vi "armctrl-arm-ctrl-exec.vi"(9 "Process Variable\nRadians":dbl, 10 "Setpoint Radians":dbl, 11 "in Linear System Loop":T1) -> (0 "Error":bool, 1 "Filtered Process\nVariable Radians":dbl, 2 "Motor Dmd":dbl, 3 "out Linear System Loop":T1)   [LabVIEW 2019]
uses:
  <vilib>/Rock Robotics/WPI/ThirdParty/JAS_Junk/TrajLib/TypeDef/LINEAR_SYSTEM_LOOP.ctl
  <vilib>/Rock Robotics/WPI/ThirdParty/JAS_Junk/TrajLib/TypeDef/LINEAR_QUADRATIC_REGULATOR.ctl
  <vilib>/Analysis/Matrix/Datatypes/RealMatrix.ctl
  <vilib>/Rock Robotics/WPI/ThirdParty/JAS_Junk/TrajLib/TypeDef/LINEAR_PLANT_INV_FF.ctl
  <vilib>/Rock Robotics/WPI/ThirdParty/JAS_Junk/TrajLib/TypeDef/KALMAN_FILTER.ctl
  <vilib>/Rock Robotics/WPI/ThirdParty/JAS_Junk/TrajLib/TypeDef/LINEAR_SYSTEM.ctl
  <vilib>/Rock Robotics/WPI/ThirdParty/JAS_Junk/TrajLib/MatBuilder_Create.vi
  <vilib>/Rock Robotics/WPI/ThirdParty/JAS_Junk/TrajLib/Trajectory_Library.lvlib
  <vilib>/Analysis/Matrix/NI_Matrix.lvlib
panel:
  # "<States,1>"
  # "<FUTURE --- CLAMP TYPE -- For now\nuse Normalize>"
  # "Steady State Gain  \n<States,Outputs>"
  # "State Estimate <Statess,1>"
  # "<States,States>"
  # "<States,Inputs>"
  # "<Outputs,States>"
  # "<Outputs,Inputs>"
  # "<States,1>"
  # "<Inputs,1>"
  # "<States,Inputs>"
  # "<States,States>"
  # "Ref State <States,1>"
  # "Comp and capped \noutput <Inputs,1>"
  # "Controller gain\n<Inputs,States>"
  # "<States,1>"
  # "<FUTURE --- CLAMP TYPE -- For now\nuse Normalize>"
  # "Steady State Gain  \n<States,Outputs>"
  # "State Estimate <Statess,1>"
  # "<States,States>"
  # "<States,Inputs>"
  # "<Outputs,States>"
  # "<Outputs,Inputs>"
  # "<States,1>"
  # "<Inputs,1>"
  # "<States,Inputs>"
  # "<States,States>"
  # "Ref State <States,1>"
  # "Comp and capped \noutput <Inputs,1>"
  # "Controller gain\n<Inputs,States>"
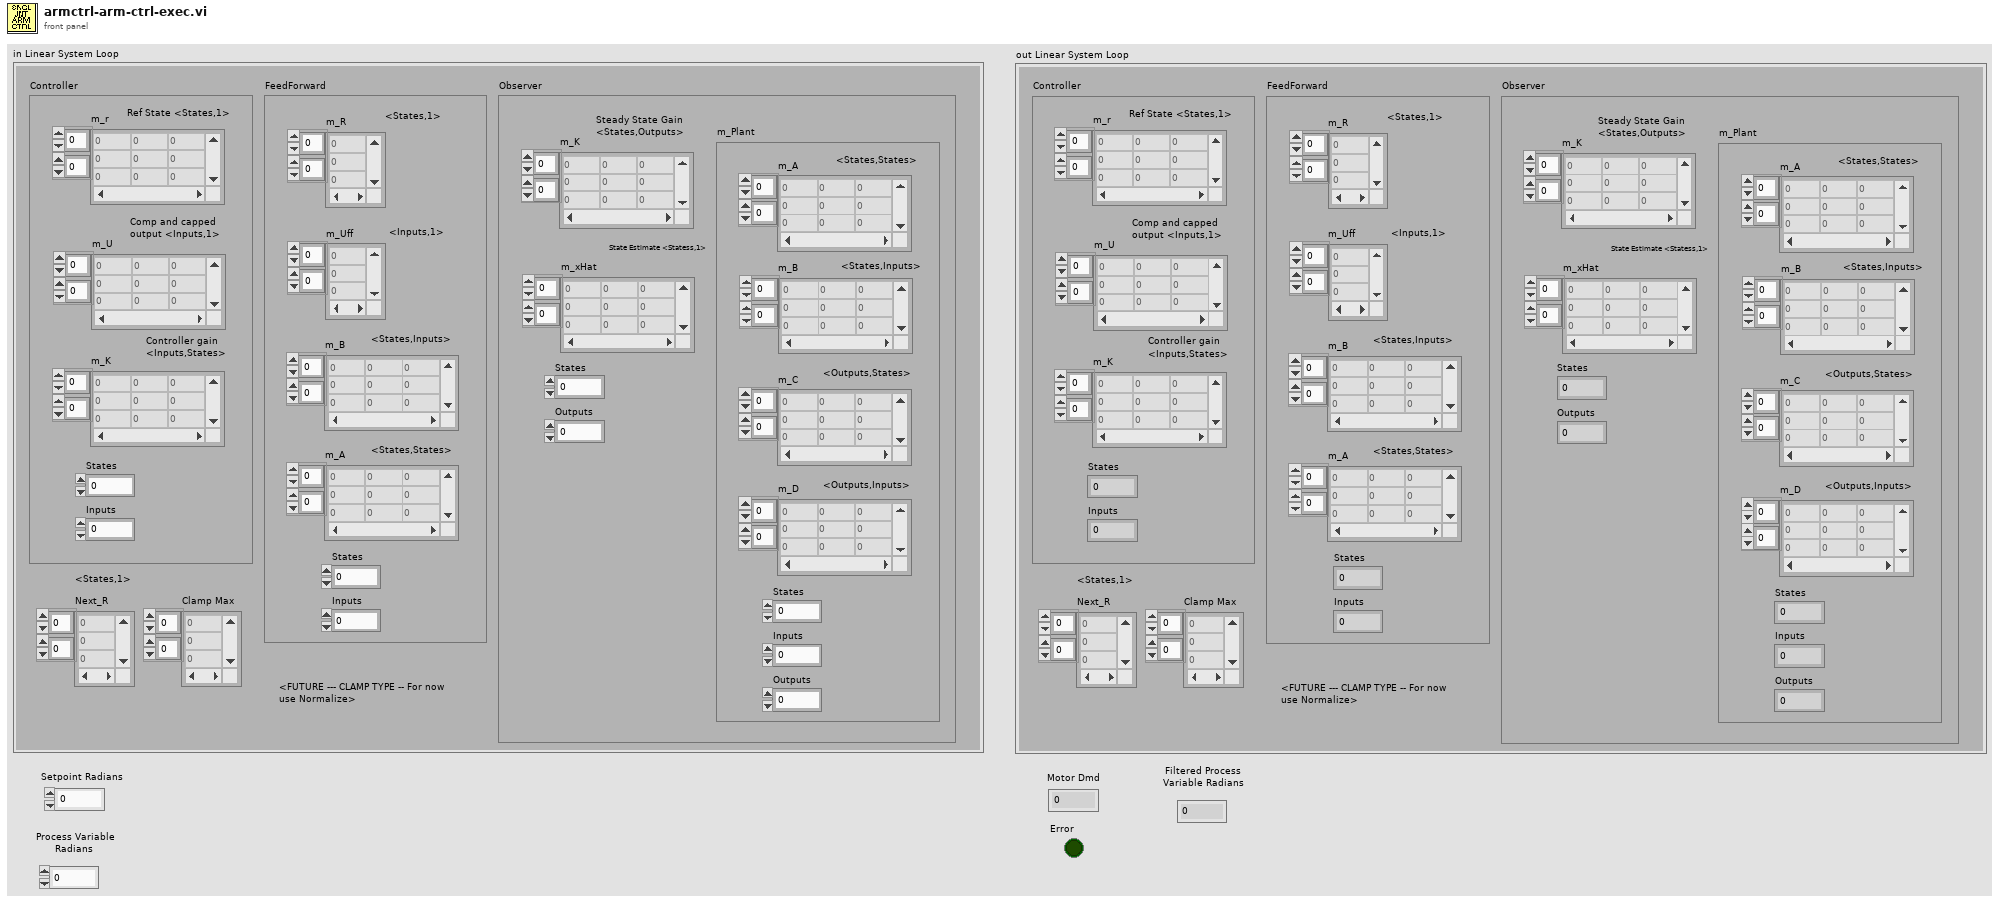
[diagram p1: front panel]
types:
  T1 = typedef "Trajectory_Library.lvlib/LINEAR_SYSTEM_LOOP.ctl" = cluster{"Controller":T2, "FeedForward":T4, "Observer":T5, "Next_R":T3, "Clamp Max":T3}
  T2 = typedef "Trajectory_Library.lvlib/LINEAR_QUADRATIC_REGULATOR.ctl" = cluster{"m_r":T3, "m_U":T3, "m_K":T3, "States":i32, "Inputs":i32}
  T3 = typedef "NI_Matrix.lvlib/RealMatrix.ctl" = dbl[][]
  T4 = typedef "Trajectory_Library.lvlib/LINEAR_PLANT_INV_FF.ctl" = cluster{"m_R":T3, "m_Uff":T3, "m_B":T3, "m_A":T3, "States":i32, "Inputs":i32}
  T5 = typedef "Trajectory_Library.lvlib/KALMAN_FILTER.ctl" = cluster{"m_K":T3, "m_xHat":T3, "States":i32, "Outputs":i32, "m_Plant":T6}
  T6 = typedef "Trajectory_Library.lvlib/LINEAR_SYSTEM.ctl" = cluster{"m_A":T3, "m_B":T3, "m_C":T3, "m_D":T3, "States":i32, "Inputs":i32, "Outputs":i32}
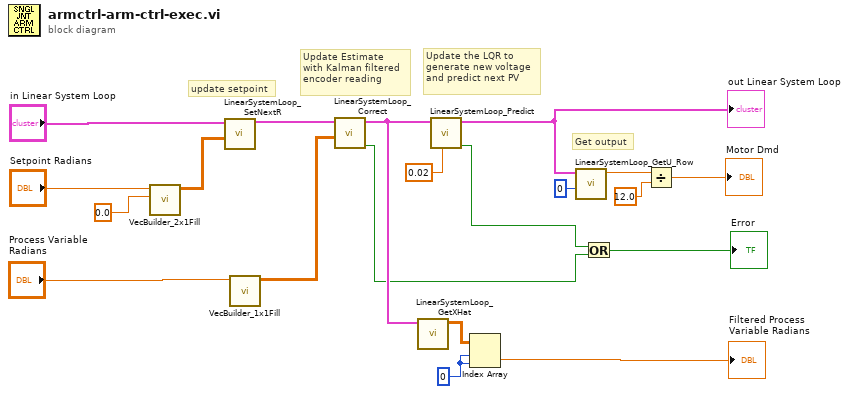
[diagram p0: block diagram]
diagram:
  w8 = 0 ("index (row)")
  # "Get output"
  # "Update the LQR to \ngenerate new voltage\nand predict next PV"
  # "update setpoint"
  # "Update Estimate\nwith Kalman filtered\nencoder reading"
  n1 = call <vilib>:"VecBuilder_2x1Fill.vi"("R1"=0.0, "R0"="Setpoint Radians") -> ("output matrix"=w19:T3)  [unwired: 9 in]
  n2 = call <vilib>:"LinearSystemLoop_SetNextR.vi"("R"=w19, "input inear System Loop"="in Linear System Loop") -> ("out Linear System Loop"=w15:T1)  [unwired: 8 in, 1 out]
  n3 = call <vilib>:"VecBuilder_1x1Fill.vi"("R0_C0"="Process Variable\nRadians") -> ("output matrix"=w7:T3)  [unwired: 10 in]
  n4 = call <vilib>:"LinearSystemLoop_Correct.vi"("Y"=w7, "input inear System Loop"=w15) -> ("Error"=w5:bool, "out Linear System Loop"=w11:T1)  [unwired: 8 in]
  n5 = call <vilib>:"LinearSystemLoop_GetXHat.vi"("input inear System Loop"=w11) -> ("XHat"=w9:T3)  [unwired: 10 in]
  n6 = call <vilib>:"LinearSystemLoop_Predict.vi"("dT_Seconds"=0.02, "input inear System Loop"=w11) -> ("Error"=w6:bool, "out Linear System Loop"=w14:T1)  [unwired: 8 in]
  "out Linear System Loop" <- w14
  n7 = Index Array(array=w9, index (row)=w8, index (col)=w8) -> (element=→"Filtered Process\nVariable Radians":dbl)
  n8 = call <vilib>:"LinearSystemLoop_GetU_Row.vi"("Row"=0, "input inear System Loop"=w14) -> ("U"=w3:dbl)  [unwired: 9 in]
  n9 = Or(x=w6, y=w5) -> (x .or. y?=→"Error":bool)
  n10 = Divide(x=w3, y=12.0) -> (x/y=→"Motor Dmd":dbl)
